vi "Event Handle Loop_Close Page.vi"(8 "error in (no error)":errorcluster, 11 "QTab Class in":refnum<class "QTab Class.lvclass">) -> (0 "error out":errorcluster, 3 "QTab Class out":refnum<class "QTab Class.lvclass">)   [LabVIEW 2020, in "QTab.lvlib" / "QTab Class.lvclass"]
uses:
  QTab Class.lvclass
  QTab Class.lvclass/QTab Class.ctl
  QMenu Class/QMenu Class.lvclass
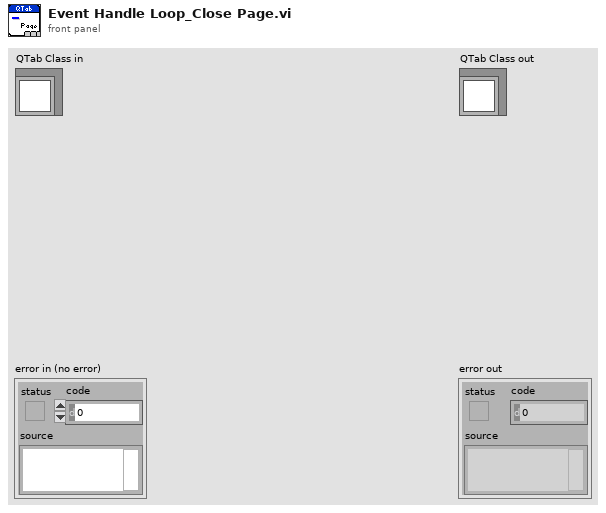
[diagram p1: front panel]
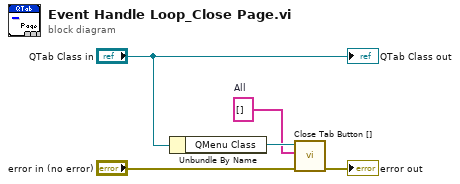
[diagram p0: block diagram]
diagram:
  w3 = string[] []  # All
  n1 = Unbundle By Name("QTab Class in") -> ("QMenu Class"=w4:refnum<class "QMenu Class.lvclass">)
  n2 = call "Close Tab Button [].vi"("error in (no error)"="error in (no error)", "Label"=w3, "QMenu Class in"=w4) -> ("error out"=→"error out":errorcluster)  [unwired: 7 in, 1 out]
  "QTab Class out" <- "QTab Class in"
